vi "Write Data.vi"(8 "error in (no error)":errorcluster, 10 "Base Data Lib:Data":refnum<class "Data.lvclass">, 11 "Generic Update Data MSG in":refnum<class "Generic Update Data MSG.lvclass">) -> (0 "error out":errorcluster, 3 "Generic Update Data MSG out":refnum<class "Generic Update Data MSG.lvclass">)   [LabVIEW 2016, in "Generic Update Data MSG.lvclass"]
uses:
  Generic Update Data MSG.lvclass
  Data/Data.lvclass
  Generic Update Data MSG.lvclass/Generic Update Data MSG.ctl
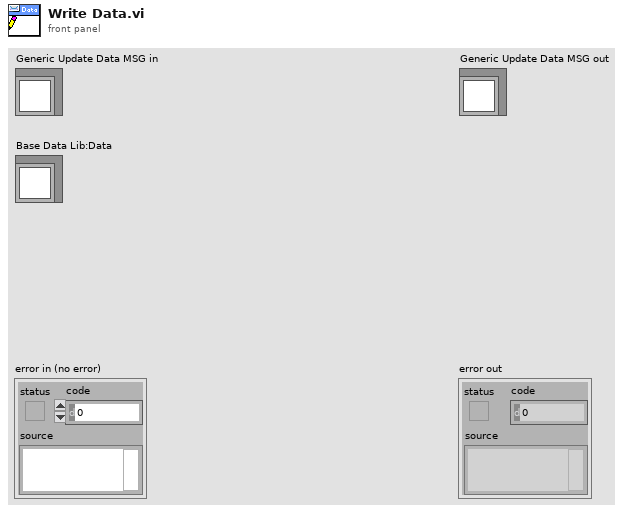
[diagram p1: front panel]
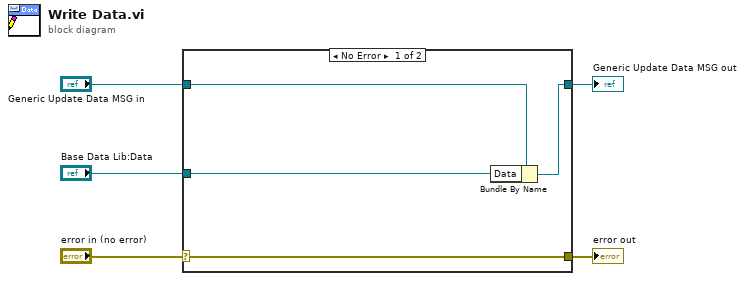
[diagram p0: block diagram]
diagram:
  n1 = case shown="No Error" "error in (no error)" {
    selector: "error in (no error)" -> [w9 w10]
    tunnel: [w9 w10] -> w4
    tunnel: [w7 w11] -> w2
    tunnel: "Generic Update Data MSG in" -> [w8 w11]
    tunnel: "Base Data Lib:Data" -> [w6 _]
    frame No Error {
      n2 = Bundle By Name(cluster=w8, "Data"=w6) -> (w7:refnum<class "Generic Update Data MSG.lvclass">)
    }
    frame Error {
    }
  }
  "error out" <- w4
  "Generic Update Data MSG out" <- w2
